vi "doc types.vi"() -> ()   [LabVIEW 2018]
uses:
  <vilib>/Utility/file.llb/Write Delimited Spreadsheet (DBL).vi
panel:
  in  "1D A":dbl[](array[numeric])
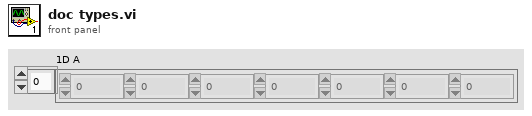
[diagram p1: front panel]
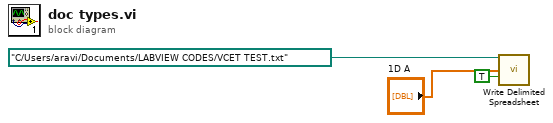
[diagram p0: block diagram]
diagram:
  n1 = call-poly <vilib>:"Write Delimited Spreadsheet.vi"("file path (dialog if empty)"=path "C:/Users/aravi/Documents/LABVIEW CODES/VCET TEST.txt", "1D data"="1D A", "append to file? (new file:F)"=TRUE) -> ()  [unwired: 11 in, 2 out]
